vi "Init_Com (SubVI).vi"() -> (3 "FindCOM":string[](array[string]), 4 "VISA Refnum out":refnum<visa-resource-name>, 6 "QueuOUT":refnum<queue>, 8 "ChannelAState":bool, 10 "ChannelBstate\nChannelBState":bool, 13 "PORT_COM":string, 14 "Com OK":bool, 15 "error out":errorcluster)   [LabVIEW 2024]
panel:
  # "Données entrante"
  # "Données sortante"
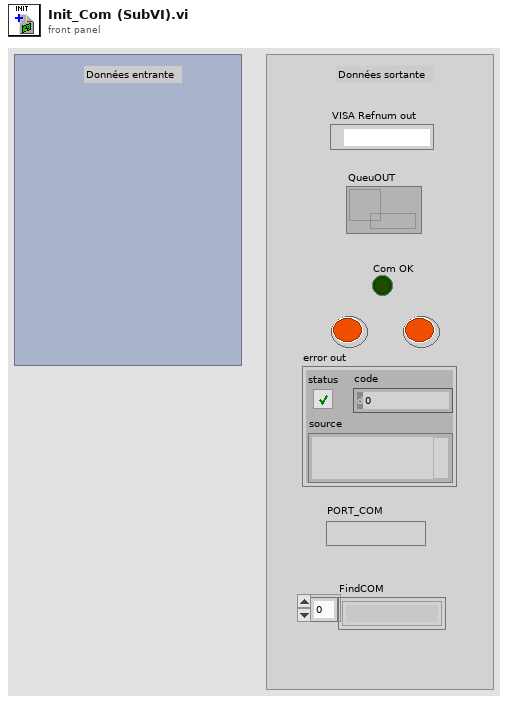
[diagram p1: front panel]
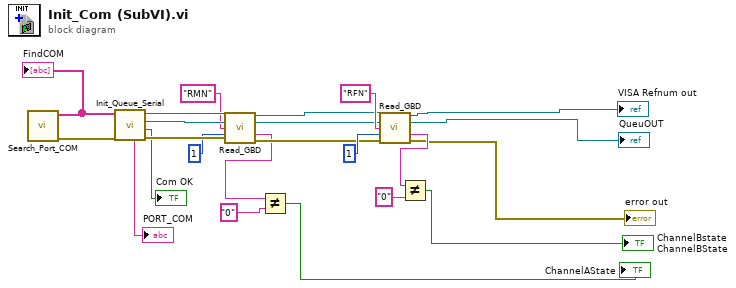
[diagram p0: block diagram]
diagram:
  n1 = call "Search_Port_COM.vi"() -> ("error out"=w1:errorcluster, "FindCOM"=w2:string[])  [unwired: 10 in]
  "FindCOM" <- w2
  n2 = call "Init_Queue_Serial.vi"("error in"=w1, "COM in"=w2) -> ("error out"=w19:errorcluster, "COM OK"=→"Com OK":bool, "queue out"=w18:refnum<queue>, "VISA Refnum out"=w20:refnum<visa-resource-name>, "COM GBF"=→"PORT_COM":string)  [unwired: 5 in]
  n3 = call "Read_GBD.vi"("VISA resource name in"=w20, "queue in"=w18, "Command"="RMN" ("string"), "byte count"=u32 1, "error in (no error)"=w19) -> ("VISA Refnum out"=w13:refnum<visa-resource-name>, "QueuOUT"=w11:refnum<queue>, "element"=w9:string, "error out"=w12:errorcluster)  [unwired: 7 in]
  n4 = Not Equal?(x=w9, y="0" ("x")) -> (x != y?=→"ChannelAState":bool)
  n5 = call "Read_GBD.vi"("VISA resource name in"=w13, "queue in"=w11, "Command"="RFN" ("string"), "byte count"=u32 1, "error in (no error)"=w12) -> ("VISA Refnum out"=→"VISA Refnum out":refnum<visa-resource-name>, "QueuOUT"=→"QueuOUT":refnum<queue>, "element"=w10:string, "error out"=→"error out":errorcluster)  [unwired: 7 in]
  n6 = Not Equal?(x=w10, y="0" ("x")) -> (x != y?=→"ChannelBstate\nChannelBState":bool)
